vi "Frame_to_word_14444A UP.vi"() -> ()   [LabVIEW 2019]
uses:
  <vilib>/addons/Modulation/Analog/support/mod_Set Error Source.vi
  <vilib>/addons/Modulation/Digital/Support/Common/Validators/mod_Generate Filter Coefficients Validate.vi
  <vilib>/addons/Modulation/Digital/General/subVIs/mod_Generate Filter Coefficients.vi
  <vilib>/addons/Modulation/Digital/General/MT Generate ASK system parameters (M).vi
  <vilib>/addons/Modulation/Analog/MT Modulate AM (DSB).vi
  <vilib>/addons/Modulation/Analog/MT Upconvert Baseband (Real).vi
  <vilib>/measure/macond.llb/IIR Filter for 1 Chan.vi
  <vilib>/express/express analysis/Spectral/Block/exnSpectralBlock spectral measurements RMS poly.vi
  <vilib>/express/express analysis/Spectral/Block/exnSpectralBlock spectral measurements RMS WFM.vi
  <vilib>/addons/Modulation/Analog/MT Downconvert Passband (Real).vi
  <vilib>/addons/Modulation/Analog/MT Demodulate AM (DSB).vi
  <vilib>/ErrorRing/Error Ring.xnode
  <vilib>/express/express analysis/Spectral/XNode/ExpressSpectralMeasurementsBlockNode.xnode
  <vilib>/addons/Modulation/niAMT.lvlib
  <vilib>/measure/NI_MAPro.lvlib
  <vilib>/addons/Modulation/niDMT.lvlib
panel:
  out "video Manchecter 9":cluster{"f0":dbl, "df":dbl, "magnitude":dbl[]}(graph)
  out "Video  2":cluster{"t0":dbl, "dt":dbl, "Y":dbl[]}(graph)
  out "Command 2":cluster{"t0":dbl, "dt":dbl, "Y":dbl[]}(graph)
  out "SOF+DATA+EOF 4":cluster{"t0":dbl, "dt":dbl, "Y":dbl[]}(graph)
  out "SOF+DATA+EOF 3":cluster{"t0":dbl, "dt":dbl, "Y":dbl[]}(graph)
  out "error out":errorcluster
  out "Array of byte":u8[](array[numeric]) format="%x"
  out "Command":cluster{"t0":dbl, "dt":dbl, "Y":dbl[]}(graph)
  out "SOF+DATA+EOF 2":cluster{"t0":dbl, "dt":dbl, "Y":dbl[]}(graph)
  out "spectrum analog signal 6":waveform(dbl)(graph)
  out "spectrum analog signal 5":cluster{"t0":dbl, "dt":dbl, "Y":dbl[]}(graph)
  out "Analog signal 8":waveform(dbl)(graph)
  out "spectrum analog signal 4":cluster{"t0":dbl, "dt":dbl, "Y":dbl[]}(graph)
  out "Analog signal 9":waveform(dbl)(graph)
  out "Analog signal 7":waveform(dbl)(graph)
  out "Analog signal 4":waveform(dbl)(graph)
  out "100% ASK":waveform(dbl)(graph)
  out "video Manchecter 8":cluster{"t0":dbl, "dt":dbl, "Y":dbl[]}(graph)
  out "video Manchecter 2":cluster{"t0":dbl, "dt":dbl, "Y":dbl[]}(graph)
  out "video Manchecter 7":waveform(dbl)(graph)
  out "video Manchecter 5":waveform(dbl)(graph)
  out "video Manchecter":cluster{"t0":dbl, "dt":dbl, "Y":dbl[]}(graph)
  in  "BIT RATE":dbl
  in  "CARRIER (hz)":dbl=13560.0
  out "Video  without CRC":cluster{"t0":dbl, "dt":dbl, "Y":dbl[]}(graph)
  out "Video":cluster{"t0":dbl, "dt":dbl, "Y":dbl[]}(graph)
  in  "LSB":u8[](array[numeric])=[80] format="%x"
  in  "MSB":u8[](array[numeric])=[178, 212, 178, 212] format="%x"
  # "App data"
  # "Protocol info"
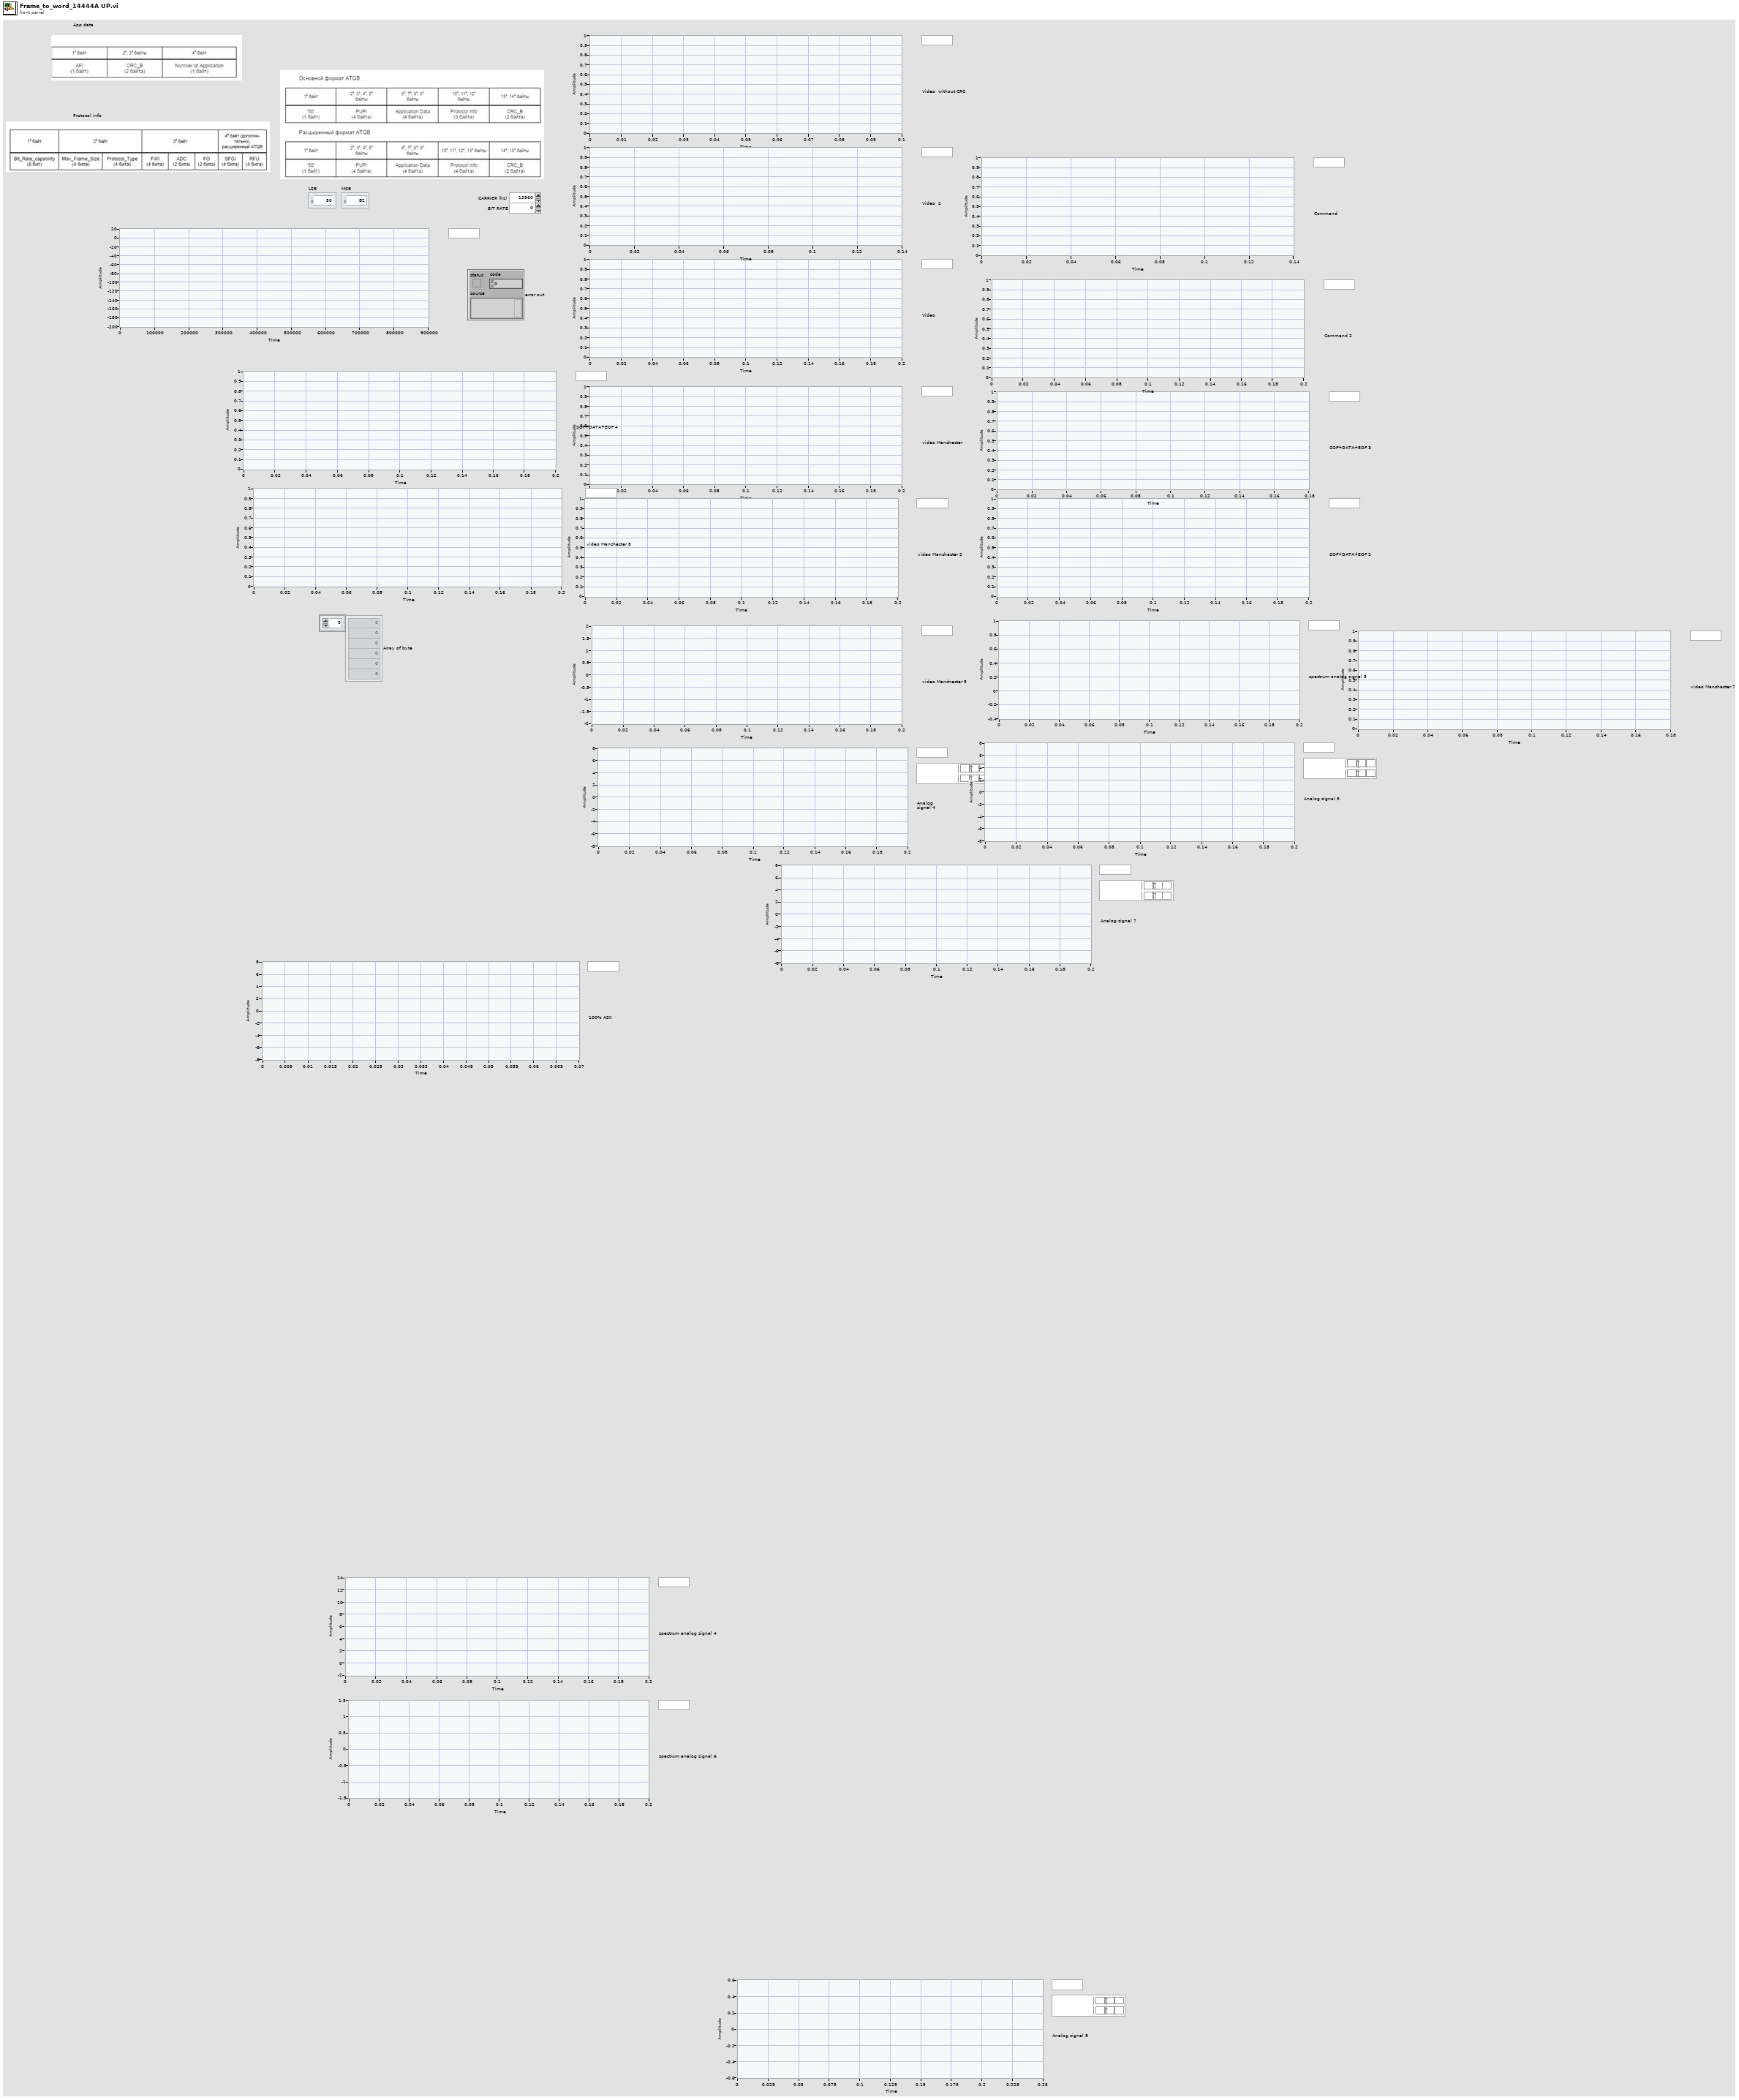
[diagram p1: front panel]
types:
  T1 = enum16{"none", "Raised Cosine", "Root Raised Cos", "Gaussian"}
  T2 = enum16{"FSK", "PSK", "QAM", "MSK", "PAM", "ASK", "CPM"}
  T3 = cluster{"Topology":enum16{"Off", "Butterworth", "Chebyshev", "Inverse Chebyshev", "Elliptic", "Bessel"}, "Type":enum16{"Lowpass", "Highpass", "Bandpass", "Bandstop"}, "Order":i32, "Lower Fc":dbl, "Upper Fc":dbl, "PB Ripple":dbl, "SB Attenuation":dbl}
  T4 = cluster{"passband ripple (dB)":dbl, "stopband start (Hz)":dbl, "stopband gain (dB)":dbl, "compute filter stopband ? (T)":bool}
  T5 = typedef "niAMT.lvlib/Complex Data Waveform.ctl" = cluster{"t0":dbl, "dt":dbl, "Y":cdb[]}
  T6 = cluster{"samples per symbol (16)":i32, "symbol map":cdb[]}
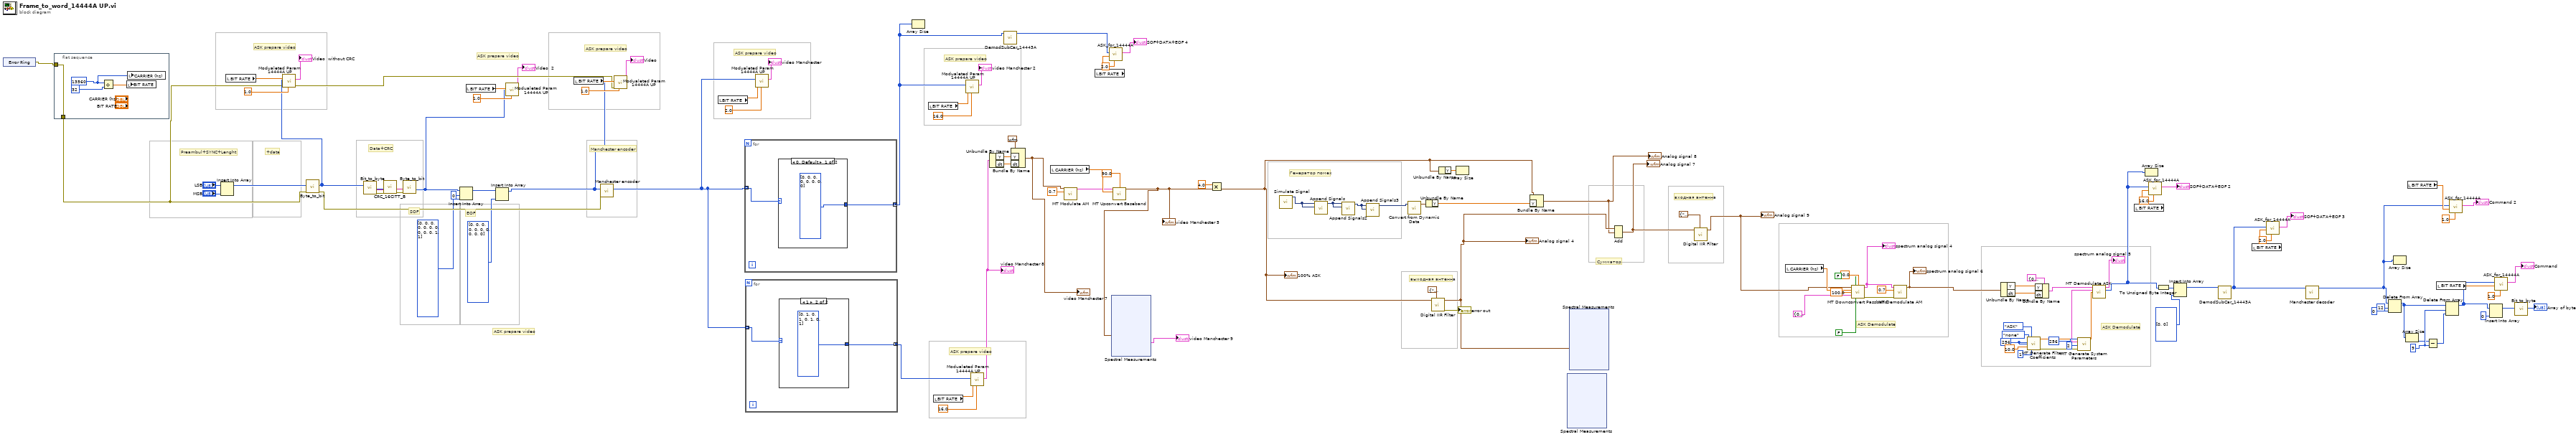
[diagram p0: block diagram]
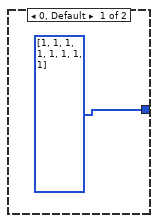
[diagram p2: hidden frame]
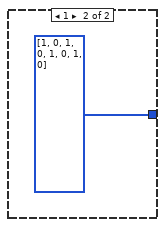
[diagram p3: hidden frame]
diagram:
  w47 = 9 ("length")
  w77 = 256 ("pulse shaping samples per symbol (16)")
  (unwired) 16.0 ("y")
  # "ASK prepare video"
  # "ASK prepare video"
  # "EOF"
  # "SOF"
  # "ASK Demodulate"
  # "ASK Demodulate"
  # "входная антенна"
  # "Сумматор"
  # "выходная антенна"
  # "Генератор помех"
  # "ASK prepare video"
  # "ASK prepare video"
  # "ASK prepare video"
  # "ASK prepare video"
  # "ASK prepare video"
  # "ASK prepare video"
  # "Manchester encoder"
  # "Data+CRC"
  # "+data"
  # "Preambul+SYNC+Lenght"
  n1 = xnode "Error Ring"() -> ("error out"=w111:errorcluster)
  n2 = flat-sequence {
    tunnel: w111 -> [w123]
    tunnel: [w123] -> w110
    frame #0 {
      w124 = u32 13560
      n3 = Divide(x=w124, y=u32 32) -> (x/y=w125:dbl)
      n4 = local write "BIT RATE"(w125) -> ()
      n5 = local write "CARRIER (hz)"(w124) -> ()
    }
  }
  n6 = Insert Into Array(array="LSB", new element="MSB") -> (w120:u8[])  [unwired: 1 in]
  n7 = local read "BIT RATE"() -> (w114:dbl)
  n8 = call "Byte_to_bit.vi"("Error In"=w110, "Array of byte"=w120) -> ("Error Out"=w112:errorcluster, "Arrray of bit"=w113:u8[])  [unwired: 5 in, 1 out]
  n9 = call "Modualeted Param 14444A UP.vi"("encoder divider"=1.0 ("y"), "Error In"=w110, "BIT RATE"=w114, "Bit stream out (NRZ encode)"=w113) -> ("Error Out"=w109:errorcluster, "output complex waveform"=→"Video  without CRC":T5)  [unwired: 6 in]
  n10 = call "Bit_to_byte.vi"("Array of bit"=w113) -> ("Error Out"=w89:errorcluster, "BYTE"=w91:string)  [unwired: 8 in, 1 out]
  n11 = call "CRC_16CITT_B.vi"("Error In"=w89, "DATA PACKET"=w91) -> ("Error Out"=w88:errorcluster, "DATA PACKET+CRC"=w90:string)  [unwired: 5 in, 1 out]
  n12 = call "Byte_to_bit.vi"("Error In"=w88, "BYTE"=w90) -> ("Arrray of bit (str)"=w4:u8[])  [unwired: 5 in, 2 out]
  n13 = Insert Into Array(array=w4, index=0, new element=u8[] [0, 0, 0, 0, 0, 0, 0, 0, 0, 0, 1, 1] ("Bit stream out (NRZ encode)")) -> (w10:u8[])
  n14 = local read "BIT RATE"() -> (w6:dbl)
  n15 = Insert Into Array(array=w10, new element=u8[] [0, 0, 0, 0, 0, 0, 0, 0, 0, 0] ("Bit stream out (NRZ encode)")) -> (w5:u8[])  [unwired: 1 in]
  n16 = call "Modualeted Param 14444A UP.vi"("encoder divider"=1.0 ("y"), "BIT RATE"=w6, "Bit stream out (NRZ encode)"=w4) -> ("output complex waveform"=→"Video  2":T5)  [unwired: 7 in, 1 out]
  n17 = local read "BIT RATE"() -> (w119:dbl)
  n18 = call "Manchester encoder.vi"("Error In"=w112, "Bit stream in"=w5) -> ("Bit stream out (Manchester encode)"=w96:u8[])  [unwired: 8 in, 1 out]
  n19 = call "Modualeted Param 14444A UP.vi"("encoder divider"=1.0 ("y"), "Error In"=w109, "BIT RATE"=w119, "Bit stream out (NRZ encode)"=w5) -> ("output complex waveform"=→"Video":T5)  [unwired: 6 in, 1 out]
  n20 = local read "BIT RATE"() -> (w107:dbl)
  n21 = for {
    tunnel: w96 -> [w128] mode=indexing
    tunnel: [w127] -> w20 mode=concatenating
    n22 = case shown="0, Default" w128 {
      tunnel: [u8[] [0, 0, 0, 0, 0, 0, 0, 0] ("output array") u8[] [1, 0, 1, 0, 1, 0, 1, 0] ("output array")] -> w127
      frame 0, Default {
      }
      frame 1 {
      }
    }
  }
  n23 = for {
    tunnel: w96 -> [w132] mode=indexing
    tunnel: [w131] -> w21 mode=concatenating
    n24 = case shown="1" w132 {
      tunnel: [u8[] [1, 1, 1, 1, 1, 1, 1, 1] ("output array") u8[] [0, 1, 0, 1, 0, 1, 0, 1] ("output array")] -> w131
      frame 0, Default {
      }
      frame 1 {
      }
    }
  }
  n25 = call "Modualeted Param 14444A UP.vi"("encoder divider"=2.0 ("y"), "BIT RATE"=w107, "Bit stream out (NRZ encode)"=w96) -> ("output complex waveform"=→"video Manchecter":T5)  [unwired: 7 in, 1 out]
  n26 = Array Size(array=w20) -> ()  [unwired: 1 out]
  n27 = local read "BIT RATE"() -> (w105:dbl)
  n28 = local read "BIT RATE"() -> (w95:dbl)
  n29 = call "Modualeted Param 14444A UP.vi"("encoder divider"=16.0 ("y"), "BIT RATE"=w105, "Bit stream out (NRZ encode)"=w20) -> ("output complex waveform"=→"video Manchecter 2":T5)  [unwired: 7 in, 1 out]
  n30 = call "Modualeted Param 14444A UP.vi"("encoder divider"=16.0 ("y"), "BIT RATE"=w95, "Bit stream out (NRZ encode)"=w21) -> ("output complex waveform"=w92:T5)  [unwired: 7 in, 1 out]
  "video Manchecter 8" <- w92
  n31 = Unbundle By Name(w92) -> ("Y"=w98:cdb[], "dt"=w97:dbl)
  n32 = call "DemodSubCar_14443A.vi"("output array"=w20) -> ("Array"=w25:u8[])  [unwired: 9 in, 1 out]
  n33 = Bundle By Name(cluster=waveform(cdb) {"t0"=timestamp(0 s since 1904-01-01), "dt"=1.0, "Y"=[]} ("waveform"), "Y"=w98, "dt"=w97) -> (w3:waveform(cdb))
  "video Manchecter 7" <- w3
  n34 = local read "CARRIER (hz)"() -> (w102:dbl)
  n35 = call-poly <vilib>:"MT Modulate AM.vi"("message signal"=w3, "modulation index"=0.7) -> ("AM modulated waveform"=w100:cluster{"t0":dbl, "dt":dbl, "Y":cdb[]})  [unwired: 12 in, 1 out]
  n36 = local read "BIT RATE"() -> (w22:dbl)
  n37 = call "ASK_for_14444A.vi"("encoder divider"=2.0 ("y"), "BIT RATE"=w22, "Bit stream out (NRZ encode)"=w25) -> ("output complex waveform"=→"SOF+DATA+EOF 4":T5)  [unwired: 7 in, 1 out]
  n38 = call-poly <vilib>:"MT Upconvert Baseband.vi"("baseband waveform (complex)"=w100, "initial phase (deg)"=90.0, "carrier frequency (Hz)"=w102) -> ("passband waveform"=w2:waveform(dbl))  [unwired: 11 in, 1 out]
  "video Manchecter 5" <- w2
  n39 = xnode "Spectral Measurements"("Signals"=w2) -> ("FFT - (RMS)"=→"video Manchecter 9":cluster{"f0":dbl, "df":dbl, "magnitude":dbl[]})  [unwired: 1 in, 2 out]
  n40 = Multiply(x=4.0, y=w2) -> (x*y=w35:waveform(dbl))
  "100% ASK" <- w35
  n41 = call "Simulate Signal"() -> ("Sine with Gaussian Noise"=w32:dynamicdata)  [unwired: 14 in, 1 out]
  n42 = call "Append Signals"("Input Signal B"=w32, "Input Signal A"=w32) -> ("Appended Signals"=w31:dynamicdata)  [unwired: 8 in, 1 out]
  n43 = call "Append Signals2"("Input Signal B"=w31, "Input Signal A"=w31) -> ("Appended Signals"=w30:dynamicdata)  [unwired: 8 in, 1 out]
  n44 = call "Append Signals3"("Input Signal B"=w30, "Input Signal A"=w30) -> ("Appended Signals"=w29:dynamicdata)  [unwired: 8 in, 1 out]
  n45 = call "Convert from Dynamic Data"("Dynamic Data Type"=w29) -> ("Waveform"=w86:waveform(dbl))  [unwired: 3 in]
  n46 = Unbundle By Name(w86) -> ("Y"=w33:dbl[])
  n47 = call-poly <vilib>:"Digital IIR Filter.vi"("IIR filter specifications"=T3 {"Topology"=enum."Butterworth", "Type"=enum."Bandpass", "Order"=3, "Lower Fc"=2000.0, "Upper Fc"=22000.0, "PB Ripple"=1.0, "SB Attenuation"=60.0}, "signal in"=w35) -> ("error out"=→"error out":errorcluster, "signal out"=w38:waveform(dbl))  [unwired: 7 in, 1 out]
  "Analog signal 4" <- w38
  n48 = Unbundle By Name(w35) -> ("Y"=w34:dbl[])
  n49 = Array Size(array=w34) -> ()  [unwired: 1 out]
  n50 = Bundle By Name(cluster=w35, "Y"=w33) -> (w37:waveform(dbl))
  "Analog signal 8" <- w37
  n51 = xnode "Spectral Measurements"() -> ()  [unwired: 2 in, 3 out]
  n52 = xnode "Spectral Measurements"("Signals"=w38) -> ()  [unwired: 1 in, 3 out]
  n53 = Add(1:w37, 2:w38) -> (0:w84:waveform(dbl))  [unwired: 1 in, 1 out]
  "Analog signal 7" <- w84
  n54 = call-poly <vilib>:"Digital IIR Filter.vi"("IIR filter specifications"=T3 {"Topology"=enum."Butterworth", "Type"=enum."Bandpass", "Order"=4, "Lower Fc"=2000.0, "Upper Fc"=22000.0, "PB Ripple"=1.0, "SB Attenuation"=60.0}, "signal in"=w84) -> ("signal out"=w64:waveform(dbl))  [unwired: 7 in, 2 out]
  "Analog signal 9" <- w64
  n55 = local read "CARRIER (hz)"() -> (w83:dbl)
  n56 = call-poly <vilib>:"MT Downconvert Passband.vi"("Waveform"=w64, "reset? (F)"=FALSE, "initial phase (deg)"=90.0, "carrier frequency (Hz)"=w83, "passband bandwidth (Hz)"=100.0, "advanced filter parameters"=T4 {"passband ripple (dB)"=0.01, "stopband start (Hz)"=0.0, "stopband gain (dB)"=-96.0, "compute filter stopband ? (T)"=TRUE}, "enable filter (T)"=FALSE) -> ("downconverted waveform (complex baseband)"=w59:T5, "error out"=w65:errorcluster)  [unwired: 5 in, 2 out]
  "spectrum analog signal 4" <- w59
  n57 = call-poly <vilib>:"MT Demodulate AM.vi"("AM modulated waveform"=w59, "modulation index"=0.7, "error in (no error)"=w65) -> ("AM demodulated waveform"=w63:waveform(dbl))  [unwired: 10 in, 2 out]
  "spectrum analog signal 6" <- w63
  n58 = Unbundle By Name(w63) -> ("Y"=w61:dbl[], "dt"=w60:dbl)
  n59 = call <vilib>:"MT Generate Filter Coefficients.vi"("pulse shaping filter (none)"=T1."none", "modulation type"=T2."ASK", "pulse shaping samples per symbol (16)"=w77, "matched samples per symbol (16)"=w77, "filter parameter"=10.0, "filter length (symbols)"=1) -> ("pulse shaping filter coefficients"=w71:dbl[], "error out"=w74:errorcluster)  [unwired: 1 in, 7 out]
  n60 = Bundle By Name(cluster=cluster{"t0":dbl, "dt":dbl, "Y":dbl[]} {"t0"=0.0, "dt"=0.0, "Y"=[]} ("AM modulated waveform"), "Y"=w61, "dt"=w60) -> (w58:cluster{"t0":dbl, "dt":dbl, "Y":dbl[]})
  n61 = call-poly <vilib>:"MT Generate System Parameters.vi"("samples per symbol (16)"=256, "M-ASK (2)"=2, "error in (no error)"=w74) -> ("ASK system parameters"=w72:T6)  [unwired: 12 out]
  n62 = call <vilib>:"MT Demodulate ASK.vi"("input complex waveform"=w58, "ASK system parameters"=w72, "matched filter coefficients"=w71) -> ("recovered complex waveform"=→"spectrum analog signal 5":T5, "output bit stream"=w16:i8[])  [unwired: 8 in, 3 out]
  n63 = local read "BIT RATE"() -> (w55:dbl)
  n64 = Array Size(array=w16) -> ()  [unwired: 1 out]
  n65 = call "ASK_for_14444A.vi"("encoder divider"=16.0 ("y"), "BIT RATE"=w55, "Bit stream out (NRZ encode)"=w16) -> ("output complex waveform"=→"SOF+DATA+EOF 2":T5)  [unwired: 7 in, 1 out]
  n66 = To Unsigned Byte Integer(number=w16) -> (unsigned 8bit integer=w19:u8[])
  n67 = Insert Into Array(array=w19, new element=u8[] [0, 0]) -> (w17:u8[])  [unwired: 1 in]
  n68 = call "DemodSubCar_14443A.vi"("output array"=w17) -> ("Array"=w15:u8[])  [unwired: 9 in, 1 out]
  n69 = local read "BIT RATE"() -> (w28:dbl)
  n70 = call "ASK_for_14444A.vi"("encoder divider"=2.0 ("y"), "BIT RATE"=w28, "Bit stream out (NRZ encode)"=w15) -> ("output complex waveform"=→"SOF+DATA+EOF 3":T5)  [unwired: 7 in, 1 out]
  n71 = call "Manchester decoder.vi"("Bit stream in"=w15) -> ("Array"=w14:u8[])  [unwired: 9 in, 1 out]
  n72 = Delete From Array(array=w14, length=12, index=0) -> (array with subset deleted=w49:u8[])  [unwired: 1 out]
  n73 = Array Size(array=w14) -> ()  [unwired: 1 out]
  n74 = Array Size(array=w49) -> (size(s)=w45:i32)
  n75 = local read "BIT RATE"() -> (w54:dbl)
  n76 = Subtract(x=w45, y=w47) -> (x-y=w46:i32)
  n77 = local read "BIT RATE"() -> (w50:dbl)
  n78 = Delete From Array(array=w49, length=w47, index=w46) -> (array with subset deleted=w43:u8[])  [unwired: 1 out]
  n79 = call "ASK_for_14444A.vi"("encoder divider"=1.0 ("y"), "BIT RATE"=w54, "Bit stream out (NRZ encode)"=w14) -> ("output complex waveform"=→"Command 2":T5)  [unwired: 7 in, 1 out]
  n80 = Insert Into Array(array=w43, new element=u8 0 ("new element/subarray")) -> (w41:u8[])  [unwired: 1 in]
  n81 = call "ASK_for_14444A.vi"("encoder divider"=1.0 ("y"), "BIT RATE"=w50, "Bit stream out (NRZ encode)"=w43) -> ("output complex waveform"=→"Command":T5)  [unwired: 7 in, 1 out]
  n82 = call "Bit_to_byte.vi"("Array of bit"=w41) -> ("Array of byte"=→"Array of byte":u8[])  [unwired: 8 in, 2 out]
